vi "Identify Node as Path.vi"(8 "error in (no error)":errorcluster, 11 "Picture Ring in":refnum<class "Node Value.lvclass">) -> (0 "error out":errorcluster, 3 "Picture Ring out":refnum<class "Node Value.lvclass">)   [LabVIEW 2019, in "Node Value.lvclass"]
uses:
  Node Value.lvclass
  Node Value.lvclass/Node Value.ctl
  Node Type--enum.ctl
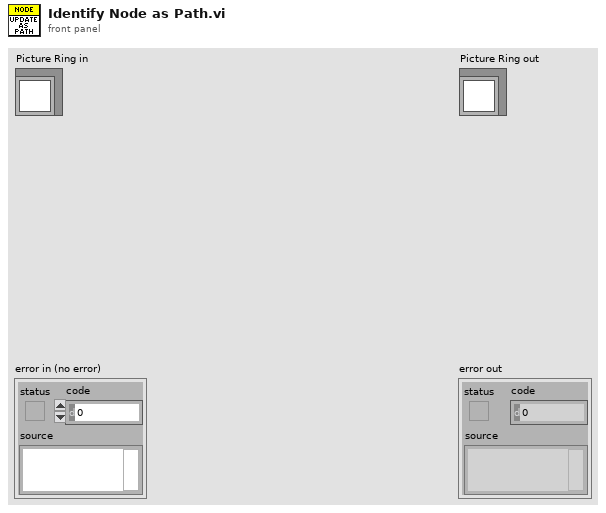
[diagram p1: front panel]
types:
  T1 = typedef "Node Value.lvclass/Node Type--enum.ctl" = enum16{"Empty", "Blocked", "Start", "End", "Path"}
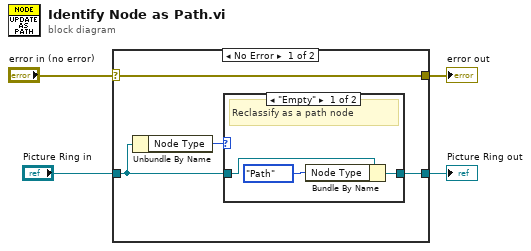
[diagram p0: block diagram]
diagram:
  n1 = case shown="No Error" "error in (no error)" {
    selector: "error in (no error)" -> [w8 w14]
    tunnel: [w8 w14] -> w3
    tunnel: [w7 w13] -> w1
    tunnel: "Picture Ring in" -> [w6 w13]
    frame No Error {
      n2 = Unbundle By Name(w6) -> ("Node Type"=w5:T1)
      n3 = case shown="\"Empty\"" w5 {
        tunnel: [w11 w12] -> w7
        tunnel: w6 -> [w9 w12]
        frame "Empty" {
          # "Reclassify as a path node"
          n4 = Bundle By Name(cluster=w9, "Node Type"=Node_Type--enum."Path") -> (w11:refnum<class "Node Value.lvclass">)
        }
        frame Default {
          # "No modifications"
        }
      }
    }
    frame Error {
    }
  }
  "error out" <- w3
  "Picture Ring out" <- w1
